vi "SwissSPAD Live_Saving Tasks Description.vi"(8 "Error In":errorcluster, 11 "Array of Saving Tasks Information":T1[](array[typedef])) -> (0 "Error Out":errorcluster, 1 "Description":string)   [LabVIEW 2021]
uses:
  SwissSPAD Live_File Saving Task Information.ctl
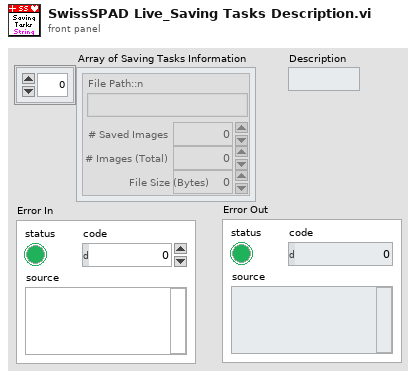
[diagram p1: front panel]
types:
  T1 = typedef "SwissSPAD Live_File Saving Task Information.ctl" = cluster{"File Path::n":string, "# Saved Images":i32, "# Images (Total)":i32, "File Size (Bytes)":i64}
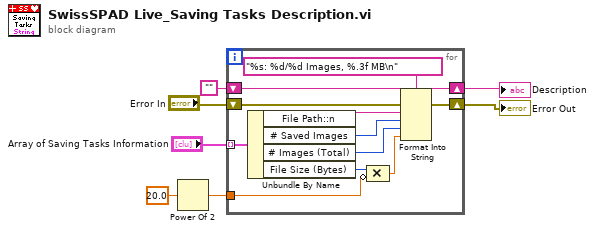
[diagram p0: block diagram]
diagram:
  n1 = Power Of 2(x=20.0) -> (2^x=w4:dbl)
  n2 = for {
    tunnel: "Array of Saving Tasks Information" -> [w19] mode=indexing
    shift-right: [w13] -> w2
    shift-left: "Error In" -> [w17]
    tunnel: w4 -> [w11]
    shift-right: [w9] -> w3
    shift-left: "" -> [w8]
    n3 = Unbundle By Name(w19) -> ("File Path::n"=w18:string, "# Saved Images"=w16:i32, "# Images (Total)"=w15:i32, "File Size (Bytes)"=w14:i64)
    n4 = Compound Arithmetic op=MULTIPLY(w14, invert w11) -> (w12:dbl)
    n5 = Format Into String(format string="%s: %d/%d Images, %.3f MB\n", initial string=w8, error in=w17, w18, w16, w15, w12) -> (resulting string=w9:string, error out=w13:errorcluster)
  }
  "Description" <- w3
  "Error Out" <- w2
